vi "log.list.vi"() -> ()   [LabVIEW 2023, in "log.lvlib"]
uses:
  log.lvlib
panel:
  out "log.list":string[][](array[string])
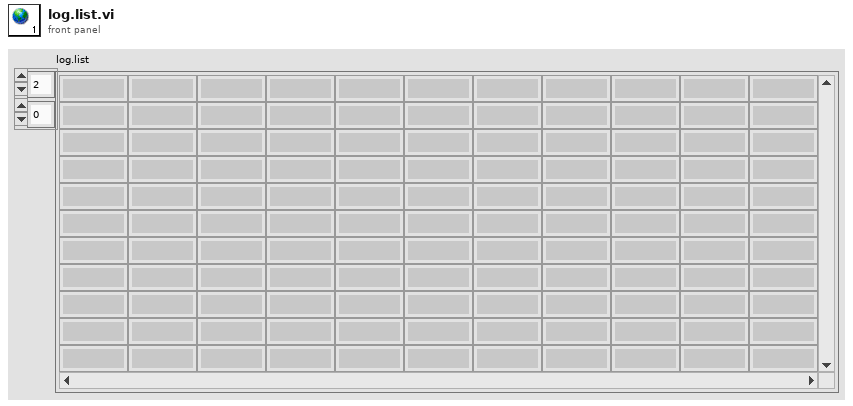
[diagram p1: front panel]
diagram:
